vi "port-odor cluster refnum split (sub-vi).vi"(8 "error in (no error)":errorcluster, 11 "port-odor and color cluster refnum":refnum<vi>) -> (0 "error out":errorcluster, 2 "element refnum cluster":T1, 3 "port-odor and color cluster refnum out":refnum<vi>)   [LabVIEW 2021]
uses:
  type-defs/port-odor with color cluster (type def).ctl
  type-defs/port-odor ring (type def).ctl
  type-defs/odor color (type def).ctl
panel:
  in  "port-odor and color cluster":T2={"port-odor ring"=0, "odor color"=9} {"port-odor ring" items=["off"]}
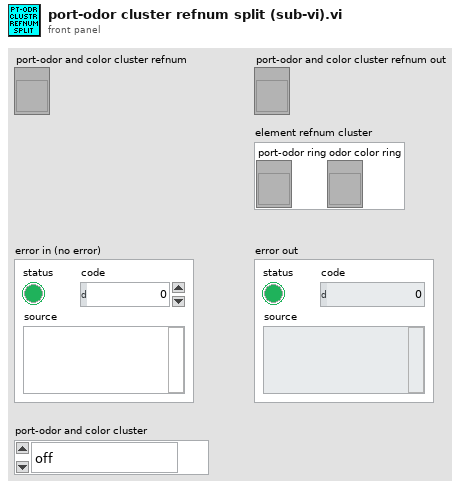
[diagram p1: front panel]
types:
  T1 = cluster{"port-odor ring":refnum<vi>, "odor color ring":refnum<vi>}
  T2 = typedef "port-odor with color cluster (type def).ctl" = cluster{"port-odor ring":T3, "odor color":T4}
  T3 = typedef "port-odor ring (type def).ctl" = u16
  T4 = typedef "odor color (type def).ctl" = u16
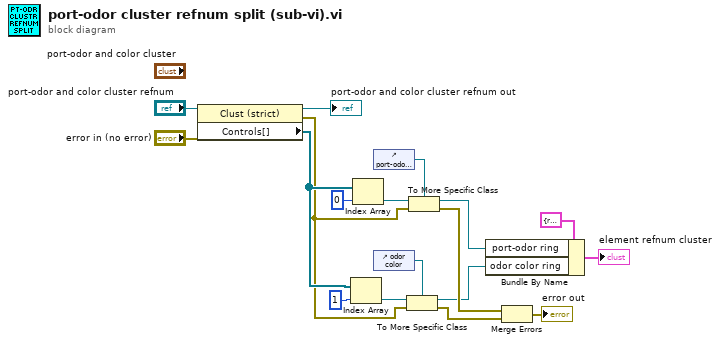
[diagram p0: block diagram]
diagram:
  n1 = property class="Clust (strict)"(reference="port-odor and color cluster refnum", error in="error in (no error)") -> (reference out=→"port-odor and color cluster refnum out":refnum<vi>, error out=w8:errorcluster, "Controls[]"=w14:refnum<vi>[])
  n2 = Index Array(array=w14, index=1) -> (element=w11:refnum<vi>)
  n3 = Index Array(array=w14, index=0) -> (element=w12:refnum<vi>)
  n4 = control-ref of="port-odor ring"() -> (w13:refnum<vi>)
  n5 = control-ref of="odor color"() -> (w10:refnum<vi>)
  n6 = To More Specific Class(target class=w10, reference=w11, error in=w8) -> (specific class reference=w3:refnum<vi>, error out=w6:errorcluster)
  n7 = To More Specific Class(target class=w13, reference=w12, error in=w8) -> (specific class reference=w4:refnum<vi>, error out=w7:errorcluster)
  n8 = Bundle By Name(cluster=T1 {"port-odor ring"=refnum, "odor color ring"=refnum} ("element refnum cluster"), "port-odor ring"=w4, "odor color ring"=w3) -> (→"element refnum cluster":T1)
  n9 = Merge Errors(w7, w6) -> (→"error out":errorcluster)
